vi "IntuitiveSteering_Y.vi"(0 "Input":dbl, 1 "Flap":dbl, 2 "Flap Saturation":dbl, 5 "Forward Time":dbl, 7 "Phase Shift":dbl, 9 "Max. Amplitude":dbl, 11 "nonZeroPositionIndex":i8) -> (4 "Servo Position":T1)   [LabVIEW 2013]
uses:
  My Computer/Controls/Servo Position.ctl
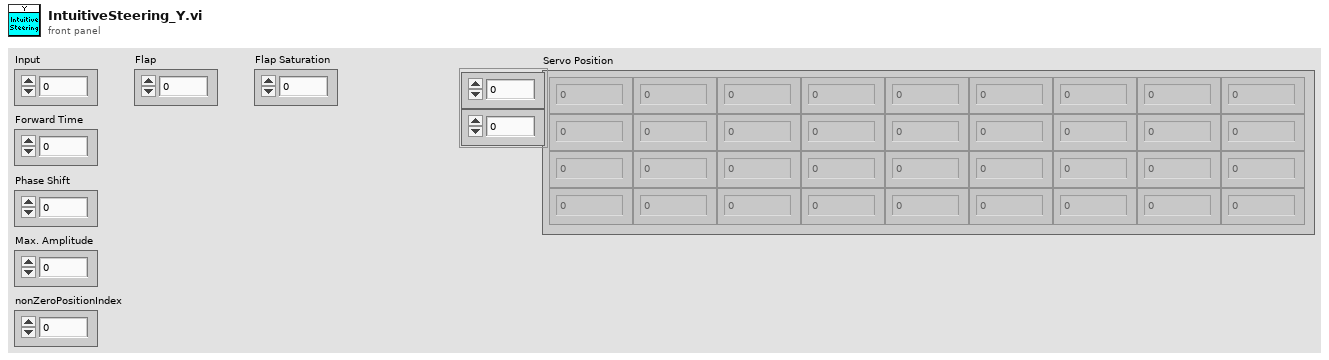
[diagram p1: front panel]
types:
  T1 = typedef "Servo Position.ctl" = dbl[][]
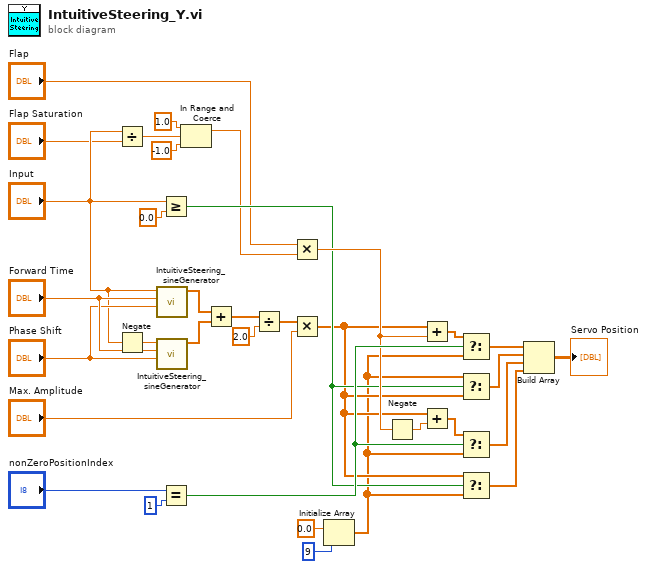
[diagram p0: block diagram]
diagram:
  n1 = Divide(x="Input", y="Flap Saturation") -> (x/y=w5:dbl)
  n2 = Negate(x="Input") -> (-x=w34:dbl)
  n3 = call "IntuitiveSteering_sineGenerator.vi"("Phase Shift"="Phase Shift", "Forward Time"="Forward Time", "Input"="Input") -> ("Fin Position"=w32:dbl[])  [unwired: 8 in]
  n4 = call "IntuitiveSteering_sineGenerator.vi"("Phase Shift"="Phase Shift", "Forward Time"="Forward Time", "Input"=w34) -> ("Fin Position"=w31:dbl[])  [unwired: 8 in]
  n5 = Greater Or Equal?(x="Input", y=0.0) -> (x >= y?=w17:bool)
  n6 = Equal?(x="nonZeroPositionIndex", y=i8 1) -> (x = y?=w25:bool)
  n7 = In Range and Coerce(upper limit=1.0, x=w5, lower limit=-1.0) -> (coerced(x)=w2:dbl)  [unwired: 1 out]
  n8 = Add(x=w32, y=w31) -> (x+y=w29:dbl[])
  n9 = Divide(x=w29, y=2.0) -> (x/y=w21:dbl[])
  n10 = Multiply(x="Flap", y=w2) -> (x*y=w18:dbl)
  n11 = Multiply(x=w21, y="Max. Amplitude") -> (x*y=w16:dbl[])
  n12 = Initialize Array(0.0 ("element"), 9 ("dimension size")) -> (w9:dbl[])
  n13 = Negate(x=w18) -> (-x=w19:dbl)
  n14 = Add(x=w16, y=w18) -> (x+y=w24:dbl[])
  n15 = Add(x=w16, y=w19) -> (x+y=w23:dbl[])
  n16 = Select(t=w24, s=w25, f=w9) -> (s? t:f=w15:dbl[])
  n17 = Select(t=w9, s=w17, f=w16) -> (s? t:f=w14:dbl[])
  n18 = Select(t=w23, s=w25, f=w9) -> (s? t:f=w13:dbl[])
  n19 = Select(t=w16, s=w17, f=w9) -> (s? t:f=w12:dbl[])
  n20 = Build Array(w15, w14, w13, w12) -> (→"Servo Position":dbl[][])
